vi "DecorateTable.vi"(6 "Elapsed Time":dbl, 7 "Current Temperature":dbl, 8 "error in (no error)":errorcluster, 9 "Current Program":dbl, 10 "Tbl Refnum":refnum<vi>, 11 "RampTable":string[][](array[string])) -> (0 "error out":errorcluster)   [LabVIEW 2013]
doc: "Use this template to build a VI to use as a subVI."
uses:
  <vilib>/Utility/miscctls.llb/LVRowAndColumnTypeDef.ctl
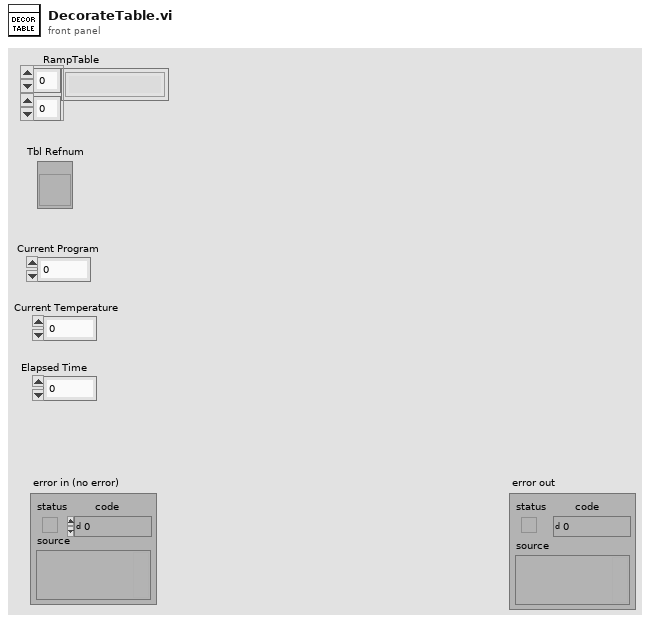
[diagram p1: front panel]
types:
  T1 = typedef "LVRowAndColumnTypeDef.ctl" = cluster{"Row":i32, "Column":i32}
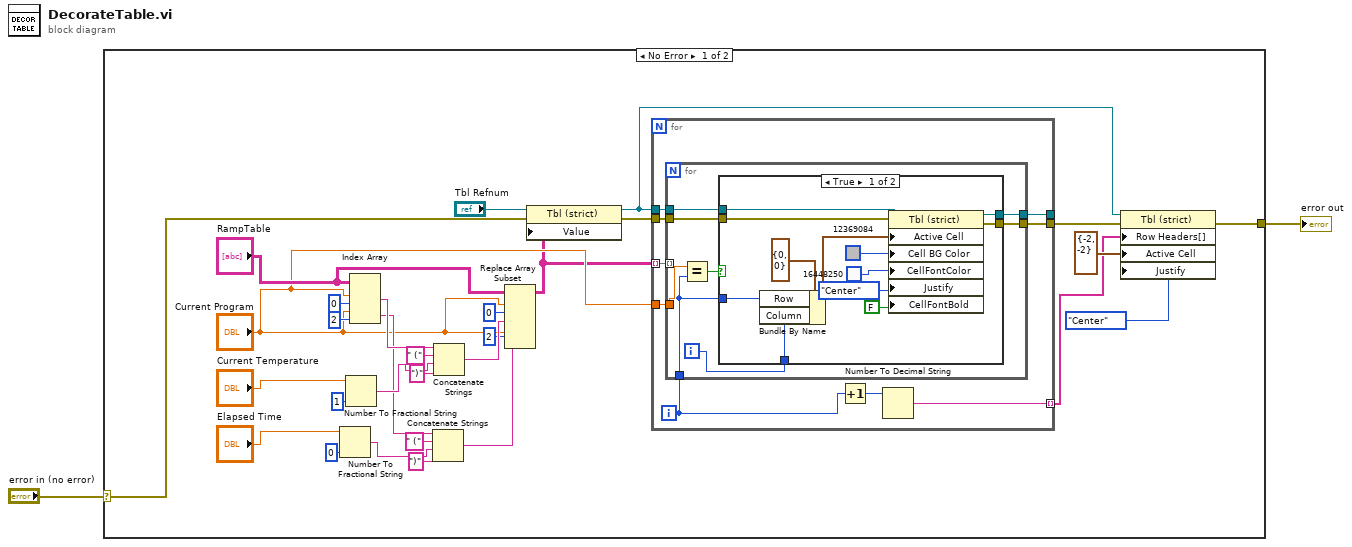
[diagram p0: block diagram]
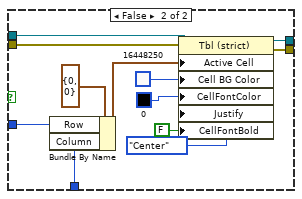
[diagram p2: hidden frame]
diagram:
  n1 = case shown="No Error" "error in (no error)" {
    selector: "error in (no error)" -> [w11 w74]
    tunnel: [w8 w74] -> w1
    frame No Error {
      n2 = Number To Fractional String(number="Elapsed Time", precision (6)=i16 0) -> (F-format string=w16:string)  [unwired: 2 in]
      n3 = Number To Fractional String(number="Current Temperature", precision (6)=i16 1) -> (F-format string=w25:string)  [unwired: 2 in]
      n4 = Index Array(array="RampTable", index (row) #1="Current Program", index (col) #1=0 ("disabled index (col)"), index (row) #2="Current Program", index (col) #2=2 ("disabled index (col)")) -> (element #1=w29:string, element #2=w18:string)
      n5 = Concatenate Strings(w18, " (" ("string"), w16, ")" ("string")) -> (w13:string)
      n6 = Concatenate Strings(w29, " (" ("string"), w25, ")" ("string")) -> (w21:string)
      n7 = Replace Array Subset(array="RampTable", new element #1=w21, index (row) #1="Current Program", index (col) #1=0 ("disabled index (col)"), new element #2=w13, index (row) #2="Current Program", index (col) #2=2 ("disabled index (col)")) -> (w5:string[][])
      n8 = property class="Tbl (strict)"(reference="Tbl Refnum", error in=w11, "Value"=w5) -> (reference out=w3:refnum<vi>, error out=w12:errorcluster)
      n9 = for {
        tunnel: w3 -> [w41]
        tunnel: w12 -> [w40]
        tunnel: [w37] -> w9
        tunnel: "Current Program" -> [w39]
        tunnel: w5 -> [w38] mode=indexing
        tunnel: [w34] -> _
        tunnel: [w33] -> w4 mode=indexing
        i -> [w35]
        n10 = for {
          tunnel: w41 -> [w49]
          tunnel: w40 -> [w48]
          tunnel: [w47] -> w37
          tunnel: w39 -> [w45]
          tunnel: w38 -> [_] mode=indexing
          tunnel: w35 -> [w43]
          tunnel: [w42] -> w34
          i -> [w46]
          n11 = Equal?(x=w45, y=w43) -> (x = y?=w44:bool)
          n12 = case shown="True" w44 {
            tunnel: w49 -> [w61 w73]
            tunnel: w48 -> [w60 w72]
            tunnel: [w59 w71] -> w47
            tunnel: w46 -> [w57 w69]
            tunnel: w43 -> [w53 w65]
            tunnel: [w50 w62] -> w42
            frame True {
              n13 = Bundle By Name(cluster=T1 {"Row"=0, "Column"=0} ("Active Cell:Active Cell"), "Row"=w53, "Column"=w57) -> (w56:T1)
              n14 = property class="Tbl (strict)"(reference=w61, error in=w60, "Active Cell"=w56, "Cell BG Color"=u32 12369084 ("Color"), "CellFontColor"=u32 16448250 ("Color"), "Justify"=enum16{"Left", "Center", "Right"}."Center" ("Active Cell:Cell Justification"), "CellFontBold"=FALSE ("Active Cell:Cell Font:Bold")) -> (reference out=w50:refnum<vi>, error out=w59:errorcluster)
            }
            frame False {
              n15 = Bundle By Name(cluster=T1 {"Row"=0, "Column"=0} ("Active Cell:Active Cell"), "Row"=w65, "Column"=w69) -> (w68:T1)
              n16 = property class="Tbl (strict)"(reference=w73, error in=w72, "Active Cell"=w68, "Cell BG Color"=u32 16448250 ("Color"), "CellFontColor"=u32 0 ("Color"), "Justify"=enum16{"Left", "Center", "Right"}."Center" ("Active Cell:Cell Justification"), "CellFontBold"=FALSE ("Active Cell:Cell Font:Bold")) -> (reference out=w62:refnum<vi>, error out=w71:errorcluster)
            }
          }
        }
        n17 = Increment(x=w35) -> (x+1=w36:i32)
        n18 = Number To Decimal String(number=w36) -> (decimal integer string=w33:string)  [unwired: 1 in]
      }
      n19 = property class="Tbl (strict)"(reference=w3, error in=w9, "Row Headers[]"=w4, "Active Cell"=T1 {"Row"=-2, "Column"=-2} ("Active Cell:Active Cell"), "Justify"=enum16{"Left", "Center", "Right"}."Center" ("Active Cell:Cell Justification")) -> (error out=w8:errorcluster)  [unwired: 1 out]
    }
    frame Error {
    }
  }
  "error out" <- w1
